vi "split_cmd_U64.vi"(9 "command":u64) -> (0 "arg2":u64, 1 "arg1":u8, 3 "name":enum8{"init", "cout", "trigwait"}(ring))   [LabVIEW 2019]
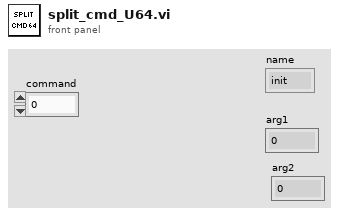
[diagram p1: front panel]
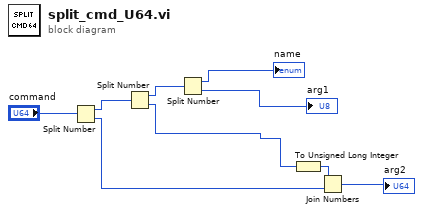
[diagram p0: block diagram]
diagram:
  n1 = Split Number(x="command") -> (hi(x)=w7:u32, lo(x)=w6:u32)
  n2 = Split Number(x=w7) -> (hi(x)=w5:u16, lo(x)=w1:u16)
  n3 = Split Number(x=w5) -> (hi(x)=→"name":u8, lo(x)=→"arg1":u8)
  n4 = To Unsigned Long Integer(number=w1) -> (unsigned 32bit integer=w3:u32)
  n5 = Join Numbers(hi=w3, lo=w6) -> ((hi.lo)=→"arg2":u64)
